vi "uTTA_OpenCOM.vi"(8 "error in":errorcluster, 10 "Log Serial Monitor(T)":bool=TRUE, 11 "VISA in":refnum<visa-resource-name>) -> (0 "error out":errorcluster, 2 "Identity":string, 3 "VISA out":refnum<visa-resource-name>)   [LabVIEW 2021]
uses:
  Serial_Port/uTTA_GV_Serial_Monitor.vi
  <vilib>/Instr/_visa.llb/VISA Configure Serial Port (Instr).vi
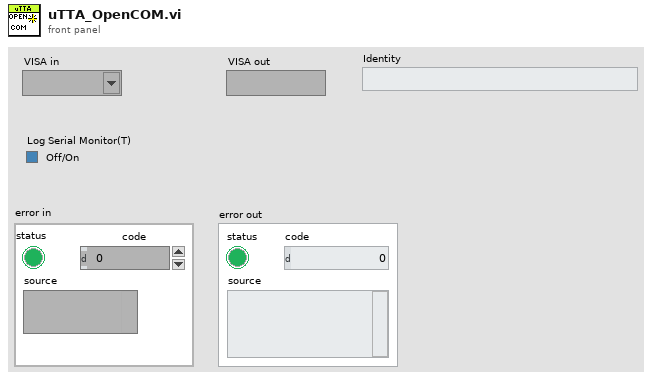
[diagram p1: front panel]
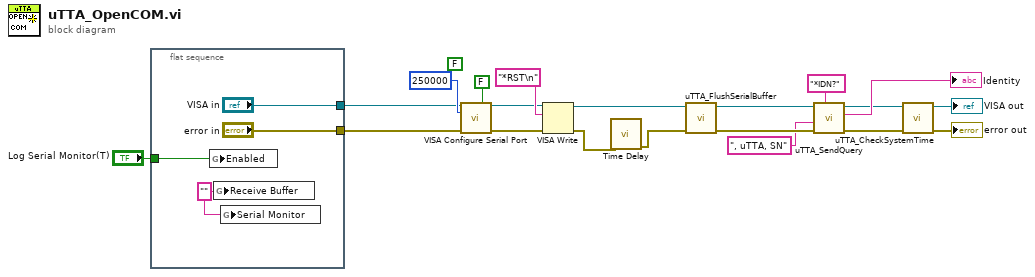
[diagram p0: block diagram]
diagram:
  (unwired) FALSE ("Enable Termination\nChar (T)")
  n1 = flat-sequence {
    tunnel: ["VISA in"] -> w14
    tunnel: ["error in"] -> w13
    tunnel: "Log Serial Monitor(T)" -> [w22]
    frame #0 {
      w21 = "" ("Serial Monitor")
      n2 = global write "uTTA_GV_Serial_Monitor.vi" "Enabled"(w22) -> ()
      n3 = global write "uTTA_GV_Serial_Monitor.vi" "Receive Buffer"(w21) -> ()
      n4 = global write "uTTA_GV_Serial_Monitor.vi" "Serial Monitor"(w21) -> ()
    }
  }
  n5 = call-poly "VISA Configure Serial Port"("VISA resource name"=w14, "Enable Termination\nChar (T)"=FALSE ("Enable Termination\nChar (T)"), "baud rate (9600)"=u32 250000, "error in (no error)"=w13) -> ("VISA resource name out"=w17:refnum<visa-resource-name>, "error out"=w18:errorcluster)  [unwired: 10 in]
  n6 = VISA Write(VISA resource name=w17, write buffer="*RST\n", error in (no error)=w18) -> (VISA resource name out=w9:refnum<visa-resource-name>, error out=w20:errorcluster)  [unwired: 1 out]
  n7 = call "Time Delay"("error in (no error)"=w20) -> ("error out"=w7:errorcluster)  [unwired: 10 in]
  n8 = call "uTTA_FlushSerialBuffer.vi"("error in (no error)"=w7, "VISA Refnum in"=w9) -> ("error out"=w6:errorcluster, "VISA Refnum out"=w8:refnum<visa-resource-name>)  [unwired: 4 in]
  n9 = call "uTTA_SendQuery.vi"("Send String"="*IDN?" ("write buffer"), "error in (no error)"=w6, "Response Qualifier(\"\")"=", uTTA, SN" ("Response Qualifier(\"\")"), "VISA Refnum in"=w8) -> ("error out"=w3:errorcluster, "Received"=→"Identity":string, "VISA Refnum out"=w4:refnum<visa-resource-name>)  [unwired: 5 in]
  n10 = call "uTTA_CheckSystemTime.vi"("error in"=w3, "VISA in"=w4) -> ("error out"=→"error out":errorcluster, "VISA Refnum out"=→"VISA out":refnum<visa-resource-name>)  [unwired: 4 in]
